vi "Measurement Logic.vi"(8 "error in":errorcluster, 9 "measurement configuration":T3={"double array in"=[3.4, 5.6], "double in"=1.2, "U32 array in"=[32, 33], "U32 in"=32, "U64 array in"=[64, 65], "U64 in"=64, "I32 array in"=[-32, -33], "I32 in"=-32, "I64 array in"=[-64, -65], "I64 in"=-64, "bool in"=TRUE, "string in"="Lorem ipsum dolor sit", "u32 color ring in"=1, "u32 animal enum in"=enum."Gopher", "DUT Pin"=""} {"u32 color ring in" items=["Red", "Green", "Blue"]}, 10 "measure call context in":refnum<class "Measure Call Context.lvclass">) -> (0 "error out":errorcluster, 1 "measurement results":T1={"xy data out"={"x_data"=[], "y_data"=[]}, "double array out"=[0.0], "double out"=0.0, "U32 array out"=[0], "U32 out"=0, "U64 array out"=[0], "U64 out"=0, "I32 array out"=[0], "I32 out"=0, "I64 array out"=[0], "I64 out"=0, "bool out"=FALSE, "string out"="Empty", "u32 color ring out"=0, "u32 animal enum out"=enum."Rabbit"} {"u32 color ring out" items=["Red", "Green", "Blue"]}, 2 "measure call context out":refnum<class "Measure Call Context.lvclass">)   [LabVIEW 2025, in "PinmapDemo.lvclass"]
doc: "Contains the core logic for executing the measurement."
uses:
  PinmapDemo.lvclass
  <vilib>/Plug-In SDKs/Measurements/Measure Call Context/Measure Call Context.lvclass
  Measurement Configuration.ctl
  Measurement Results.ctl
  <vilib>/gRPC/Generated APIs/ni/protobuf/types/RPC Messages/ni_protobuf_types_DoubleXYData.ctl
  <extravilib>/ChannelInstances/Event Messenger-bool/Instantiate.vi
  PinmapDemo.lvclass/PinmapDemo.ctl
  <vilib>/gRPC/Generated APIs/ni/protobuf/types/ni.protobuf.types.lvlib
  <vilib>/Plug-In SDKs/Measurements/Measure Call Context/Reserve Sessions - 1Pin.vi
  session-management/flexrio148x/Session Management flexrio 148x.lvlib
  <vilib>/Plug-In SDKs/Clients/Session Management V1/Session Reservation/Session Reservation.lvclass
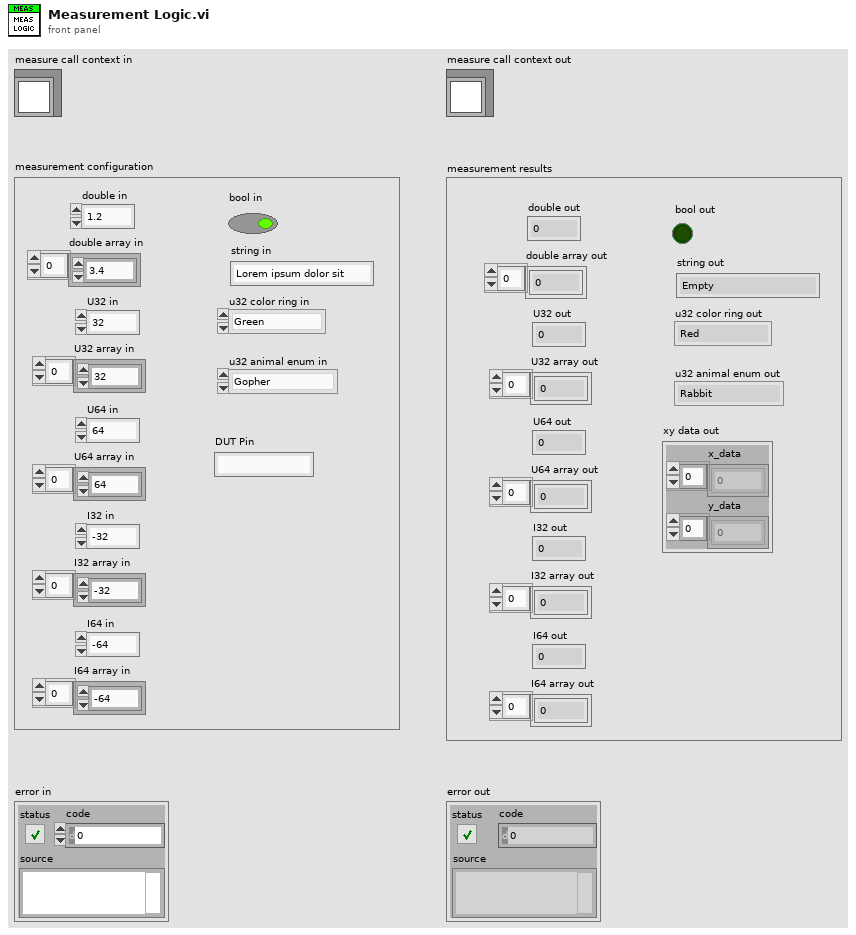
[diagram p1: front panel]
types:
  T1 = typedef "PinmapDemo.lvclass/Measurement Results.ctl" = cluster{"xy data out":T2, "double array out":dbl[], "double out":dbl, "U32 array out":u32[], "U32 out":u32, "U64 array out":u64[], "U64 out":u64, "I32 array out":i32[], "I32 out":i32, "I64 array out":i64[], "I64 out":i64, "bool out":bool, "string out":string, "u32 color ring out":u32, "u32 animal enum out":enum32{"Rabbit", "Gopher", "Badger"}}
  T2 = typedef "ni.protobuf.types.lvlib/ni_protobuf_types_DoubleXYData.ctl" = cluster{"x_data":dbl[], "y_data":dbl[]}
  T3 = typedef "PinmapDemo.lvclass/Measurement Configuration.ctl" = cluster{"double array in":dbl[], "double in":dbl, "U32 array in":u32[], "U32 in":u32, "U64 array in":u64[], "U64 in":u64, "I32 array in":i32[], "I32 in":i32, "I64 array in":i64[], "I64 in":i64, "bool in":bool, "string in":string, "u32 color ring in":u32, "u32 animal enum in":enum32{"Rabbit", "Gopher", "Badger"}, "DUT Pin":string}
  T4 = typedef "Event Messenger-bool.lvlib/))Channel.ctl" = refnum<queue>
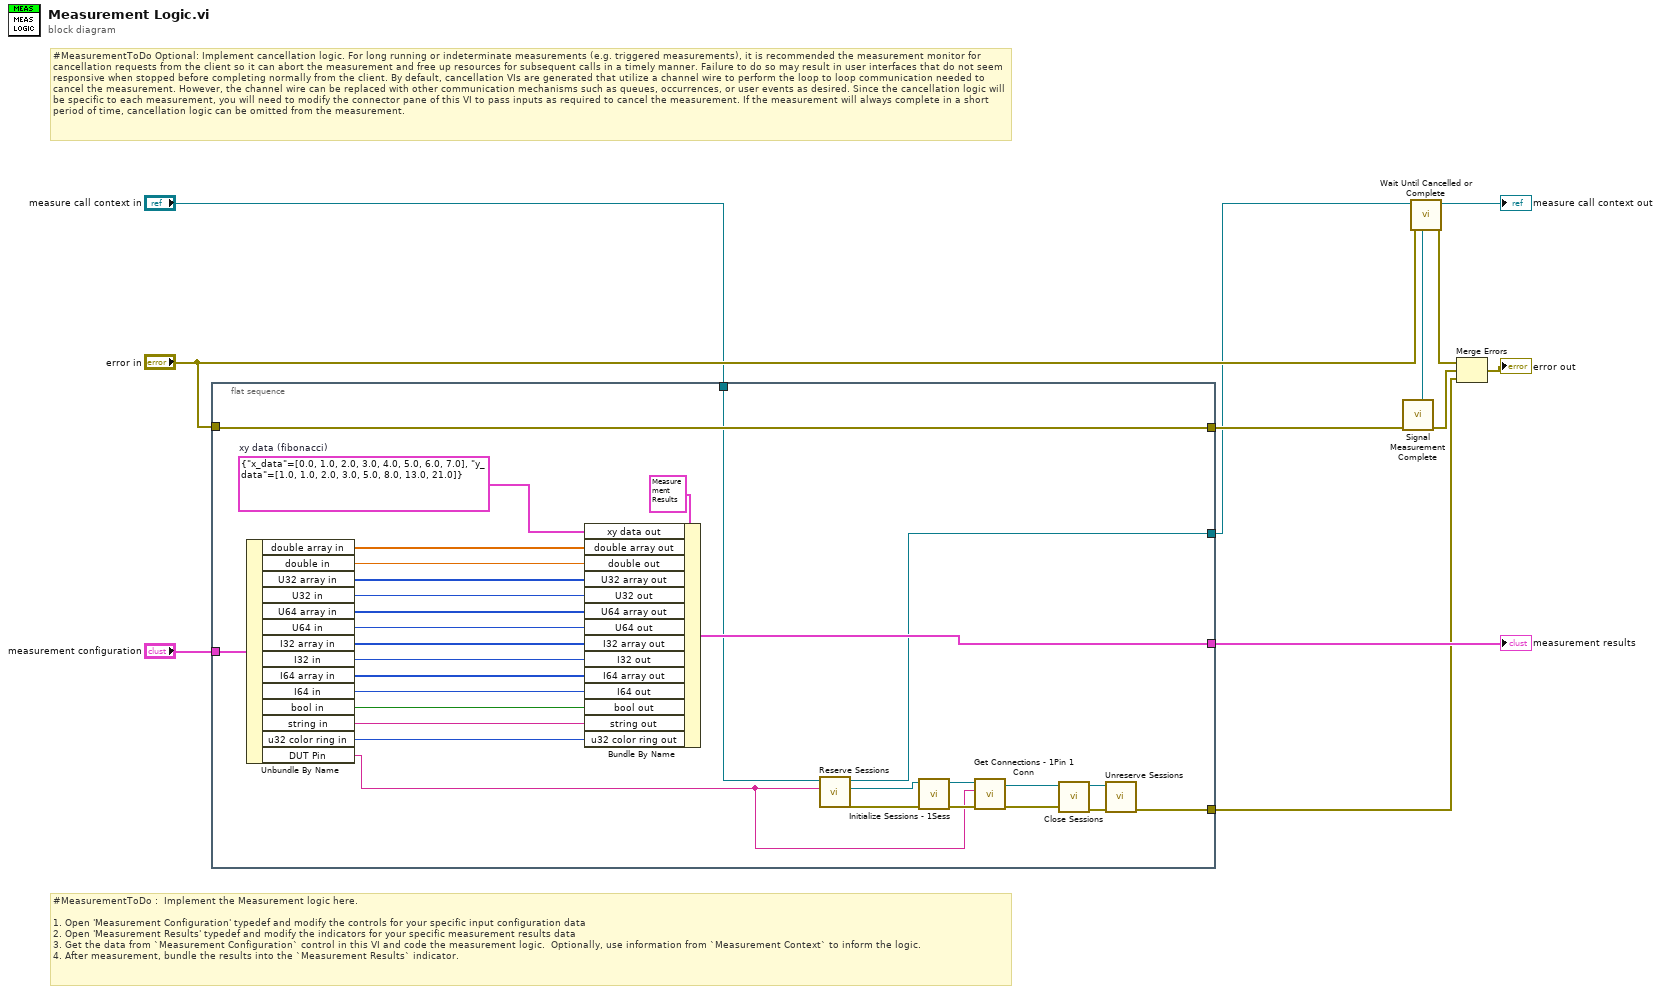
[diagram p0: block diagram]
diagram:
  # "#MeasurementToDo Optional: Implement cancellation logic. For long running or indeterminate measurements (e.g. triggered measurements), it is recommended the measurement monitor for cancellation requests from the client so it can abort the measurement and free up resources for subsequent calls in a timely manner. Failure to do so may result in user interfaces that do not seem responsive when stopped before completing normally from the client. By default, cancellation VIs are generated that utilize a channel wire to perform the loop to loop communication needed to cancel the measurement. However, the channel wire can be replaced with other communication mechanisms such as queues, occurrences, or user events as desired. Since the cancellation logic will be specific to each measurement, you will need to modify the connector pane of this VI to pass inputs as required to cancel the measurement. If the measurement will always complete in a short period of time, cancellation logic can be omitted from the measurement."
  # "#MeasurementToDo :  Implement the Measurement logic here.\n\n1. Open 'Measurement Configuration' typedef and modify the controls for your specific input configuration data\n2. Open 'Measurement Results' typedef and modify the indicators for your specific measurement results data\n3. Get the data from `Measurement Configuration` control in this VI and code the measurement logic.  Optionally, use information from `Measurement Context` to inform the logic.\n4. After measurement, bundle the results into the `Measurement Results` indicator."
  n1 = flat-sequence {
    tunnel: "measurement configuration" -> [w27]
    tunnel: [w26] -> w11
    tunnel: "error in" -> [w25]
    tunnel: [w25] -> w8
    tunnel: "measure call context in" -> [w24]
    tunnel: [w23] -> w2
    tunnel: [w13] -> w1
    frame #0 {
      w28 = T2 {"x_data"=[0.0, 1.0, 2.0, 3.0, 4.0, 5.0, 6.0, 7.0], "y_data"=[1.0, 1.0, 2.0, 3.0, 5.0, 8.0, 13.0, 21.0]}  # xy data (fibonacci)
      n2 = Unbundle By Name(w27) -> ("double array in"=w41:dbl[], "double in"=w40:dbl, "U32 array in"=w39:u32[], "U32 in"=w38:u32, "U64 array in"=w37:u64[], "U64 in"=w36:u64, "I32 array in"=w35:i32[], "I32 in"=w34:i32, "I64 array in"=w33:i64[], "I64 in"=w32:i64, "bool in"=w31:bool, "string in"=w30:string, "u32 color ring in"=w29:u32, "DUT Pin"=w18:string)
      n3 = Bundle By Name(cluster=T1 {"xy data out"={"x_data"=[], "y_data"=[]}, "double array out"=[], "double out"=0.0, "U32 array out"=[0], "U32 out"=0, "U64 array out"=[0], "U64 out"=0, "I32 array out"=[0], "I32 out"=0, "I64 array out"=[0], "I64 out"=0, "bool out"=FALSE, "string out"="Empty", "u32 color ring out"=0, "u32 animal enum out"=enum."Rabbit"} ("Measurement Results"), "xy data out"=w28, "double array out"=w41, "double out"=w40, "U32 array out"=w39, "U32 out"=w38, "U64 array out"=w37, "U64 out"=w36, "I32 array out"=w35, "I32 out"=w34, "I64 array out"=w33, "I64 out"=w32, "bool out"=w31, "string out"=w30, "u32 color ring out"=w29) -> (w26:T1)
      n4 = call-poly <vilib>:"Reserve Sessions.vi"("pin or relay name"=w18, "measurement context in"=w24) -> ("error out"=w21:errorcluster, "session reservation out"=w22:refnum<class "Session Reservation.lvclass">, "measurement context out"=w23:refnum<class "Measure Call Context.lvclass">)  [unwired: 7 in]
      n5 = call "Initialize Sessions - 1Sess.vi"("error in"=w21, "session reservation in"=w22) -> ("error out"=w20:errorcluster, "session reservation out"=w19:refnum<class "Session Reservation.lvclass">)  [unwired: 6 in, 2 out]
      n6 = call "Get Connections - 1Pin 1 Conn.vi"("error in"=w20, "pin or relay name"=w18, "session reservation in"=w19) -> ("error out"=w14:errorcluster, "session reservation out"=w15:refnum<class "Session Reservation.lvclass">)  [unwired: 6 in, 1 out]
      n7 = call <vilib>:"Close Sessions.vi"("error in"=w14, "session reservation in"=w15) -> ("error out"=w17:errorcluster, "session reservation out"=w16:refnum<class "Session Reservation.lvclass">)  [unwired: 8 in]
      n8 = call <vilib>:"Unreserve Sessions.vi"("error in"=w17, "session reservation in"=w16) -> ("error out"=w13:errorcluster)  [unwired: 9 in]
    }
  }
  n9 = call "Signal Measurement Complete.vi"("error in (no error)"=w8) -> ("error out"=w6:errorcluster, "done channel"=w7:T4)  [unwired: 9 in]
  n10 = call "Wait Until Cancelled or Complete.vi"("done channel"=w7, "error in (no error)"="error in", "measure call context in"=w2) -> ("error out"=w5:errorcluster, "measure call context out"=→"measure call context out":refnum<class "Measure Call Context.lvclass">)  [unwired: 7 in]
  n11 = Merge Errors(w5, w6, w1) -> (→"error out":errorcluster)
  "measurement results" <- w11
